vi "Global IDs.vi"() -> ()   [LabVIEW 2023, in "RFFixtureCharact.RFPM.lvlib" / "Charact Result Accessor.lvclass"]
uses:
  Charact Result Accessor.lvclass
panel:
  in  "SNP_FILE_METADATA_PREFIX":string="!National Instruments | "
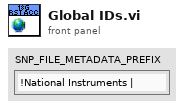
[diagram p1: front panel]
diagram:
